vi "Subvi rising edge detector.vi"(10 "Input":bool) -> (2 "Output":bool)   [LabVIEW 2017]
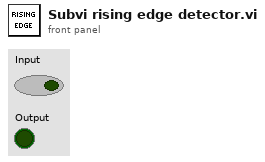
[diagram p1: front panel]
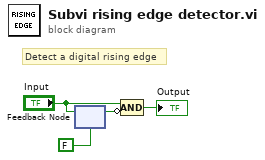
[diagram p0: block diagram]
diagram:
  # "Detect a digital rising edge"
  n1 = feedback-in #1("Input") -> ()
  n2 = feedback #1(FALSE ("Input")) -> (w3:bool)
  n3 = Compound Arithmetic op=AND("Input", invert w3) -> (→"Output":bool)
